vi "run experiment.vi"(4 "Sync Camera Acquisition":bool, 5 "Log File Name":path, 6 "Ctr Odor Pressure":dbl, 7 "Pressure Sequence (Ch 2-4)":dbl[][](array[numeric]), 8 "Valve Sequence Data":T1(array[cluster]), 9 "mixture sequence array":string[](array[string]), 10 "Time Sequence":dbl[](array[numeric]), 11 "MFCS_EZ":T2) -> (0 "Aborted?":bool)   [LabVIEW 2016]
uses:
  <userlib>/Fluigent/Fluigent MFCS/FluigentMFCS_Full.llb/_EZmfcsRefNum.ctl
  <userlib>/Fluigent/Fluigent MFCS/FluigentMFCS_Full.llb/_EZmfcsEnum.ctl
  <userlib>/Fluigent/Fluigent MFCS/FluigentMFCS_Full.llb/MFCS_EZ Write Channel Pressure.vi
  Globals/PressuresGlobal.vi
panel:
  out "Log File Name":path
  in  "stop":bool
  out "Step Time":u8(slide) scale=0.0..100.0
  out "Current State":string
  out "Remaining Time":dbl
  out "Experiment Progress":u8(slide) scale=0.0..100.0
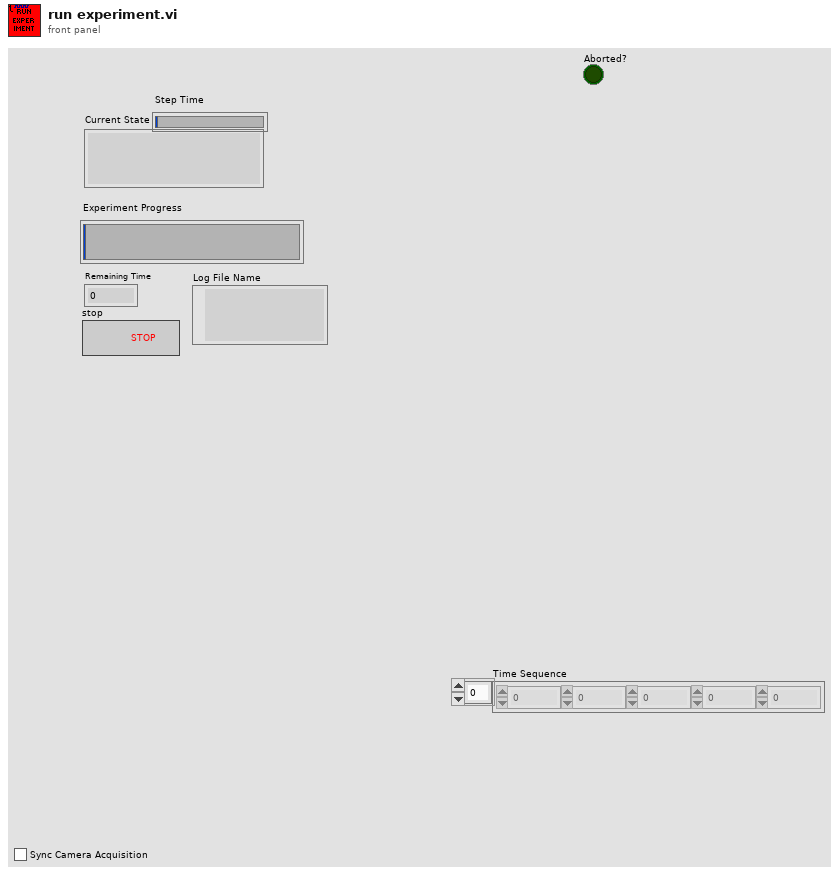
[diagram p1: front panel]
types:
  T1 = cluster{"Flowboards":enum16{"A", "B", "C"}[], "Channels":enum16{"1", "2", "3", "4", "5", "6", "7", "8"}[], "States":bool[]}[]
  T2 = typedef "_EZmfcsRefNum.ctl" = refnum<k1>
  T3 = enum16{"Release", "Create", "Send", "Wait", "Cancel"}
  T4 = cluster{"Flowboards":enum16{"A", "B", "C"}[], "Channels":enum16{"1", "2", "3", "4", "5", "6", "7", "8"}[], "States":bool[]}
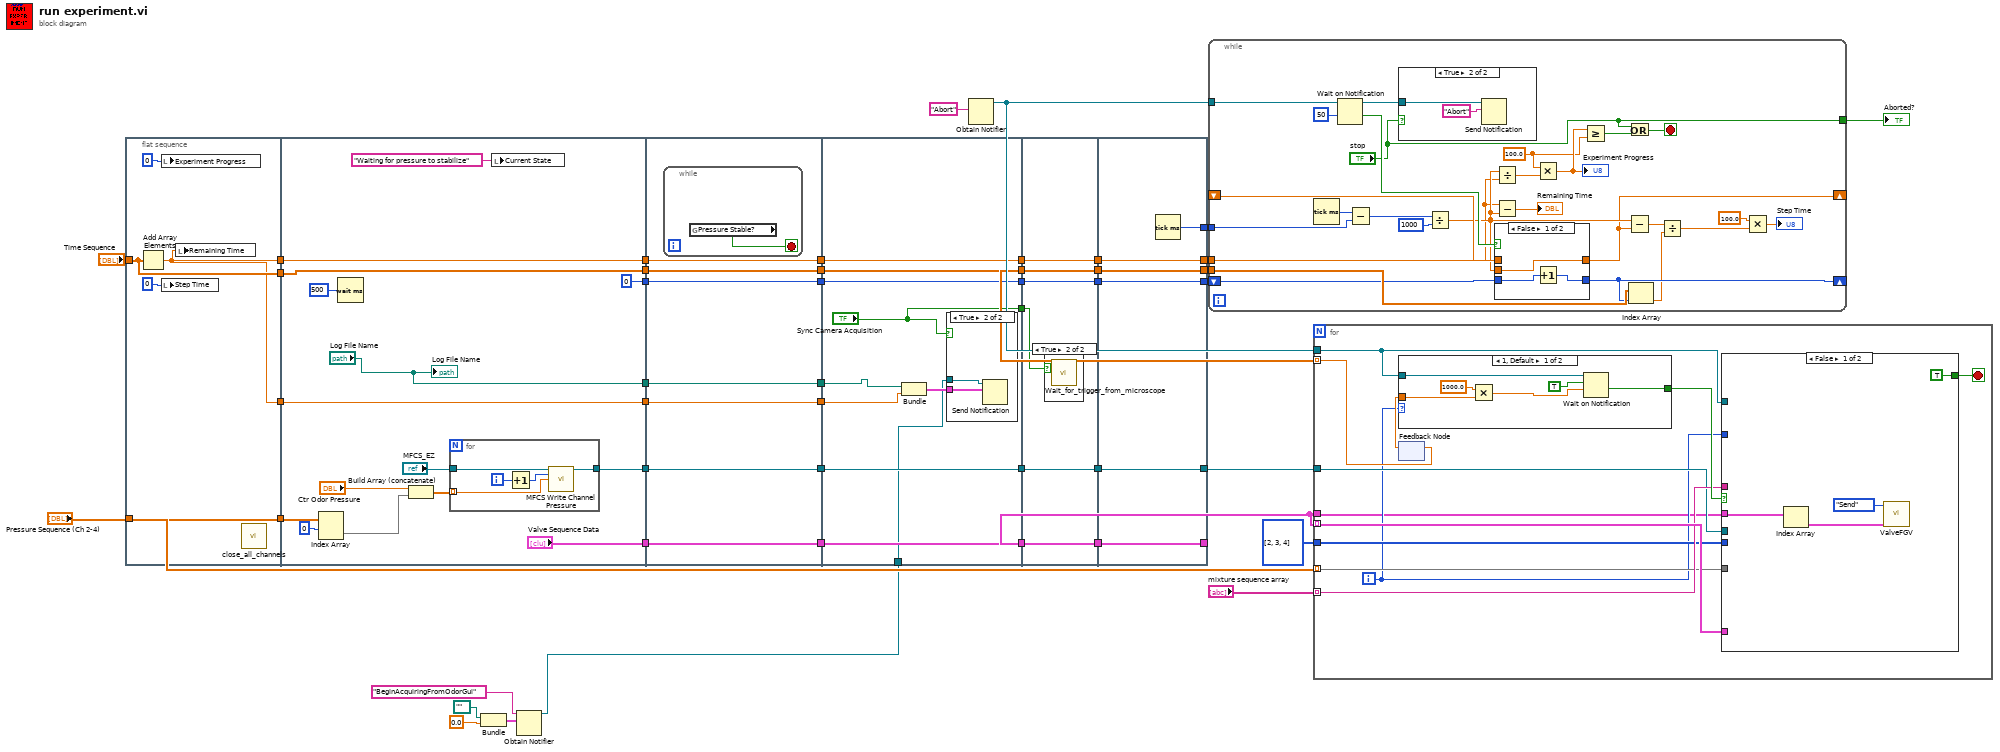
[diagram p0: block diagram]
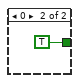
[diagram p6: hidden frame]
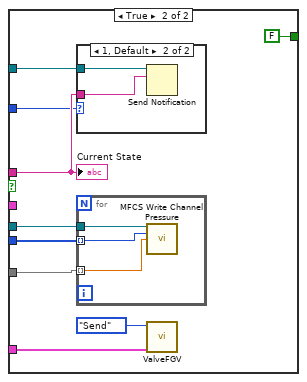
[diagram p7: hidden frame]
diagram:
  n1 = flat-sequence {
    tunnel: "Pressure Sequence (Ch 2-4)" -> [w52]
    tunnel: [w52] -> w42
    tunnel: "Time Sequence" -> [w49]
    tunnel: [w49] -> w34
    tunnel: [w48] -> w33
    tunnel: [w48] -> w14
    tunnel: w42 -> [w67]
    tunnel: [w58] -> w31
    tunnel: ["Valve Sequence Data"] -> w30
    tunnel: [0] -> w29
    tunnel: [w56] -> w28
    tunnel: [w55] -> w27
    tunnel: w34 -> [w56]
    tunnel: w33 -> [w55]
    tunnel: [w54] -> w15
    tunnel: w14 -> [w54]
    tunnel: ["Log File Name"] -> w1
    tunnel: w31 -> [w79]
    tunnel: [w79] -> w22
    tunnel: w30 -> [w78]
    tunnel: [w78] -> w21
    tunnel: w29 -> [w77]
    tunnel: [w77] -> w20
    tunnel: w28 -> [w76]
    tunnel: [w76] -> w19
    tunnel: w27 -> [w75]
    tunnel: [w75] -> w18
    tunnel: [w74] -> w16
    tunnel: w15 -> [w74]
    tunnel: [w73] -> w2
    tunnel: w1 -> [w73]
    tunnel: w22 -> [w90]
    tunnel: [w90] -> w13
    tunnel: w21 -> [w89]
    tunnel: [w89] -> w11
    tunnel: w20 -> [w88]
    tunnel: [w88] -> w9
    tunnel: w19 -> [w87]
    tunnel: [w87] -> w7
    tunnel: w18 -> [w86]
    tunnel: [w86] -> w5
    tunnel: w17 -> [w84]
    tunnel: w16 -> [w83]
    tunnel: ["Sync Camera Acquisition"] -> w3
    tunnel: w2 -> [w81]
    tunnel: w13 -> [w98]
    tunnel: [w98] -> w12
    tunnel: w11 -> [w97]
    tunnel: [w97] -> w10
    tunnel: w9 -> [w96]
    tunnel: [w96] -> w8
    tunnel: w7 -> [w95]
    tunnel: [w95] -> w6
    tunnel: w5 -> [w94]
    tunnel: [w94] -> w4
    tunnel: w3 -> [w93]
    tunnel: [w100] -> w38
    tunnel: [w101] -> w39
    tunnel: [w102] -> w40
    tunnel: [w103] -> w36
    tunnel: [w104] -> w43
    tunnel: w12 -> [w104]
    tunnel: w10 -> [w103]
    tunnel: w8 -> [w102]
    tunnel: w6 -> [w101]
    tunnel: w4 -> [w100]
    tunnel: [w99] -> w37
    frame #0 {
      n2 = Add Array Elements(numeric array=w49) -> (sum=w48:dbl)
      n3 = local write "Experiment Progress"(u8 0 ("Experiment Progress")) -> ()
      n4 = local write "Step Time"(u8 0 ("Step Time")) -> ()
      n5 = local write "Remaining Time"(w48) -> ()
      n6 = call "close_all_channels.vi"() -> ()  [unwired: 12 in]
    }
    frame #1 {
      n7 = Index Array(array=w67, index (row)=0) -> (element=w63:dbl[])  [unwired: 1 in]
      n8 = Wait (ms)(milliseconds to wait=u32 500) -> ()  [unwired: 1 out]
      n9 = Build Array (concatenate)("Ctr Odor Pressure", w63) -> (w62:dbl[])
      n10 = for {
        tunnel: "MFCS_EZ" -> [w72]
        tunnel: w62 -> [w71] mode=indexing
        tunnel: [w70] -> w58
        i -> [w69]
        n11 = Increment(x=w69) -> (x+1=w68:i32)
        n12 = call-poly <userlib>:"MFCS Write Channel Pressure.vi"("MFCS_EZ"=w72, "Channel Number (default=1)"=w68, "Pressure (mBar)"=w71) -> ("MFCS_EZ out"=w70:T2)  [unwired: 11 in, 1 out]
      }
      n13 = local write "Current State"("Waiting for pressure to stabilize" ("Current State")) -> ()
      "Log File Name" <- "Log File Name"
    }
    frame #2 {
      n14 = while {
        stop <- w80 stop-if-true
        n15 = global read "PressuresGlobal.vi" "Pressure Stable?"() -> (w80:bool)
      }
    }
    frame #3 {
      n16 = Bundle("Log File Name"=w81, "Start Water"=w83) -> (w85:cluster{"Log File Name":path, "Start Water":dbl})  [unwired: 1 in]
      n17 = case shown="True" "Sync Camera Acquisition" {
        tunnel: w84 -> [_ w92]
        tunnel: w85 -> [_ w91]
        frame False {
        }
        frame True {
          n18 = Send Notification(notification=w91, notifier=w92) -> ()  [unwired: 1 in, 2 out]
        }
      }
    }
    frame #4 {
      n19 = case shown="True" w93 {
        frame False {
        }
        frame True {
          n20 = call "Wait_for_trigger_from_microscope.vi"() -> ()  [unwired: 12 in]
        }
      }
    }
    frame #5 {
      n21 = Tick Count (ms)() -> (millisecond timer value=w99:u32)
    }
  }
  n22 = Bundle("Log File Name"=path "", 0.0) -> (w24:cluster{"Log File Name":path, dbl})  [unwired: 1 in]
  n23 = Obtain Notifier(name (unnamed)="BeginAcquiringFromOdorGui", notification data type=w24) -> (notifier out=w17:refnum<notifier>)  [unwired: 2 in, 2 out]
  n24 = Obtain Notifier(notification data type="Abort" ("notification")) -> (notifier out=w47:refnum<notifier>)  [unwired: 3 in, 2 out]
  n25 = while {
    tunnel: w47 -> [w126]
    tunnel: w38 -> [w115]
    tunnel: w37 -> [w131]
    tunnel: w39 -> [w121]
    shift-right: [w111] -> _
    shift-left: _ -> [w123]
    shift-right: [w119] -> _
    shift-left: w40 -> [w120]
    tunnel: ["stop"] -> w32
    stop <- w106 stop-if-true
    w108 = 100.0 ("x")
    n26 = Tick Count (ms)() -> (millisecond timer value=w122:u32)
    n27 = Wait on Notification(notifier=w126, timeout in ms (-1)=50) -> (notifier out=w117:refnum<notifier>, timed out?=w124:bool)  [unwired: 2 in, 2 out]
    n28 = Subtract(x=w122, y=w131) -> (x-y=w130:u32)
    n29 = case shown="True" "stop" {
      tunnel: w117 -> [_ w133]
      frame False {
      }
      frame True {
        n30 = Send Notification(notification="Abort", notifier=w133) -> ()  [unwired: 1 in, 2 out]
      }
    }
    n31 = Divide(x=w130, y=u32 1000) -> (x/y=w116:dbl)
    n32 = Divide(x=w116, y=w115) -> (x/y=w127:dbl)
    n33 = Subtract(x=w115, y=w116) -> (x-y=→"Remaining Time":dbl)
    n34 = case shown="False" w124 {
      tunnel: w116 -> [w136 _]
      tunnel: [w136 w138] -> w111
      tunnel: w123 -> [_ w138]
      tunnel: w120 -> [w135 w137]
      tunnel: [w134 w137] -> w119
      frame False {
        n35 = Increment(x=w135) -> (x+1=w134:i32)
      }
      frame True {
      }
    }
    n36 = Multiply(x=w108, y=w127) -> (x*y=w109:dbl)
    "Experiment Progress" <- w109
    n37 = Greater Or Equal?(x=w109, y=w108) -> (x >= y?=w107:bool)
    n38 = Or(x="stop", y=w107) -> (x .or. y?=w106:bool)
    n39 = Subtract(x=w116, y=w111) -> (x-y=w110:dbl)
    n40 = Index Array(array=w121, index=w119) -> (element=w118:dbl)
    n41 = Divide(x=w110, y=w118) -> (x/y=w113:dbl)
    n42 = Multiply(x=100.0, y=w113) -> (x*y=→"Step Time":dbl)
  }
  "Aborted?" <- w32
  n43 = for {
    tunnel: w47 -> [w143]
    tunnel: w39 -> [w142] mode=indexing
    tunnel: w36 -> [w149] mode=indexing
    tunnel: "mixture sequence array" -> [w148] mode=indexing
    tunnel: "Pressure Sequence (Ch 2-4)" -> [w147] mode=indexing
    tunnel: i32[] [2, 3, 4] -> [w146]
    tunnel: w43 -> [w145]
    tunnel: w36 -> [w139]
    i -> [w140]
    stop <- w144 stop-if-true
    n44 = feedback-in #1(w142) -> ()
    n45 = feedback #1() -> (w141:dbl)  [unwired: 1 in]
    n46 = case shown="1, Default" w140 {
      tunnel: w141 -> [w156 _]
      tunnel: [w153 TRUE ("timed out?")] -> w150
      tunnel: w143 -> [w151 _]
      frame 1, Default {
        n47 = Multiply(x=1000.0, y=w156) -> (x*y=w155:dbl)
        n48 = Wait on Notification(notifier=w151, ignore previous (F)=TRUE, timeout in ms (-1)=w155) -> (timed out?=w153:bool)  [unwired: 1 in, 3 out]
      }
      frame 0 {
      }
    }
    n49 = case shown="False" w150 {
      tunnel: w149 -> [_ w166]
      tunnel: w148 -> [_ w164]
      tunnel: w147 -> [_ w168]
      tunnel: w146 -> [_ w170]
      tunnel: w145 -> [_ w169]
      tunnel: w143 -> [_ w165]
      tunnel: [TRUE FALSE] -> w144
      tunnel: w140 -> [_ w162]
      tunnel: w139 -> [w159 _]
      frame False {
        n50 = Index Array(array=w159) -> (element=w158:T4)  [unwired: 1 in]
        n51 = call "ValveFGV.vi"("Valve Data"=w158, "Action"=T3."Send") -> ()  [unwired: 6 in, 4 out]
      }
      frame True {
        n52 = case shown="1, Default" w162 {
          tunnel: w165 -> [_ w172]
          tunnel: w164 -> [_ w171]
          frame 0 {
          }
          frame 1, Default {
            n53 = Send Notification(notification=w171, notifier=w172) -> ()  [unwired: 1 in, 2 out]
          }
        }
        n54 = for {
          tunnel: w170 -> [w175] mode=indexing
          tunnel: w169 -> [w174]
          tunnel: w168 -> [w173] mode=indexing
          n55 = call-poly <userlib>:"MFCS Write Channel Pressure.vi"("MFCS_EZ"=w174, "Channel Number (default=1)"=w175, "Pressure (mBar)"=w173) -> ()  [unwired: 11 in, 2 out]
        }
        n56 = call "ValveFGV.vi"("Valve Data"=w166, "Action"=T3."Send") -> ()  [unwired: 6 in, 4 out]
        "Current State" <- w164
      }
    }
  }
